vi "Generate XML String with Parser API.vi"() -> ()   [LabVIEW 2023]
doc: "This example illustrates how to create an XML document and save it as an XML file."
uses:
  <vilib>/Analysis/baseanly.llb/Mean (DBL).vi
  <vilib>/xml/Close Reference(Node).vi
  <resource>/objmgr/DOMUserDefRef.rc
  <vilib>/xml/NI_XML.lvlib
  <vilib>/Analysis/NI_AALBase.lvlib
panel:
  out "Generated XML":string
  # "Overview: Demonstrates the use of the XML Parser VIs and functions to generate an XML string that can adhere to an arbitrary schema.\nInstructions:\nRun the VI."
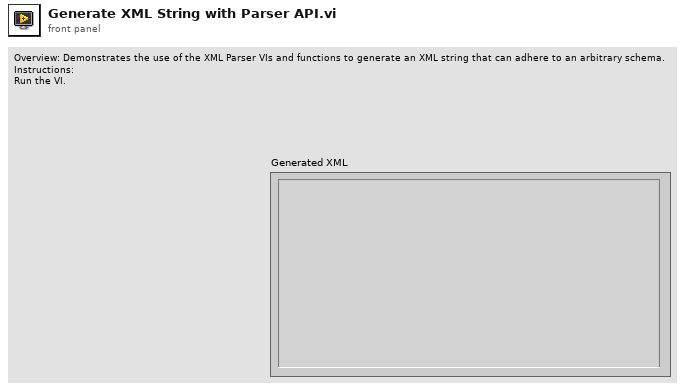
[diagram p1: front panel]
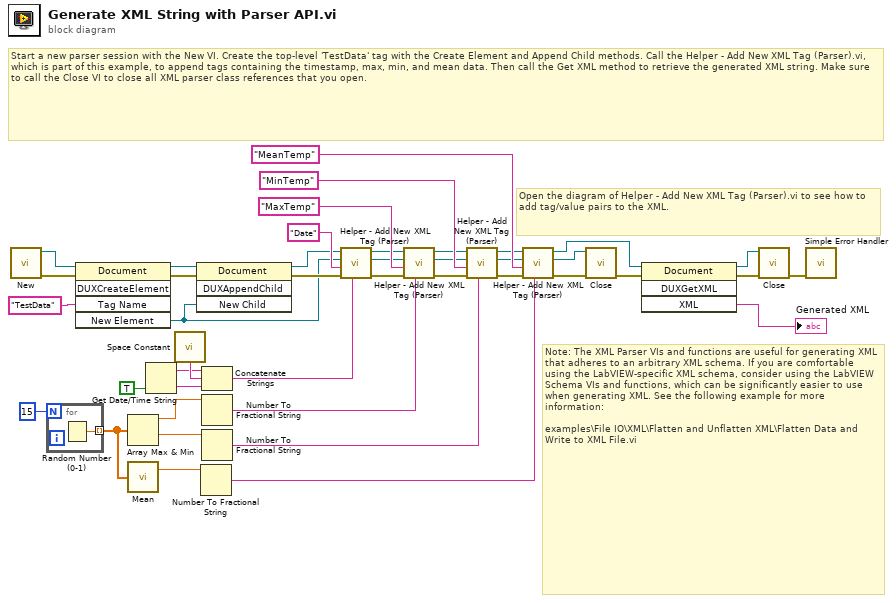
[diagram p0: block diagram]
diagram:
  # "Note: The XML Parser VIs and functions are useful for generating XML that adheres to an arbitrary XML schema. If you are comfortable using the LabVIEW-specific XML schema, consider using the LabVIEW Schema VIs and functions, which can be significantly easier to use when generating XML. See the following example for more information:\n\nexamples\\File IO\\XML\\Flatten and Unflatten XML\\Flatten Data and Write to XML File.vi"
  # "Open the diagram of Helper - Add New XML Tag (Parser).vi to see how to add tag/value pairs to the XML."
  # "Start a new parser session with the New VI. Create the top-level 'TestData' tag with the Create Element and Append Child methods. Call the Helper - Add New XML Tag (Parser).vi, which is part of this example, to append tags containing the timestamp, max, min, and mean data. Then call the Get XML method to retrieve the generated XML string. Make sure to call the Close VI to close all XML parser class references that you open."
  n1 = call <vilib>:"New.vi"() -> ("error out"=w29:errorcluster, "DOM document out"=w26:refnum<k20>)  [unwired: 1 in, 7 out]
  n2 = for {
    N: 15 -> [_]
    tunnel: [w43] -> w34 mode=indexing
    n3 = Random Number (0-1)() -> (number: 0 to 1=w43:dbl)
  }
  n4 = invoke class="Document" method="DUXCreateElement"(reference=w26, error in=w29, "Tag Name"="TestData" ("Qualified Name")) -> (reference out=w30:refnum<k20>, error out=w28:errorcluster, "New Element"=w5:refnum<k20>)  [unwired: 2 in, 2 out]
  n5 = Array Max & Min ("Max & Min")(array=w34) -> (max value=w1:dbl, min value=w2:dbl)  [unwired: 2 out]
  n6 = call-poly <vilib>:"Mean.vi"("X"=w34) -> ("mean"=w32:dbl)  [unwired: 1 out]
  n7 = Get Date/Time String(want seconds? (F)=TRUE) -> (date string=w40:string, time string=w39:string)  [unwired: 2 out]
  n8 = call <vilib>:"Space Constant.vi"() -> ("String"=w41:string)
  n9 = invoke class="Document" method="DUXAppendChild"(reference=w30, error in=w28, "New Child"=w5) -> (reference out=w9:refnum<k20>, error out=w7:errorcluster)  [unwired: 1 in, 2 out]
  n10 = Number To Fractional String(number=w32) -> (F-format string=w22:string)  [unwired: 3 out]
  n11 = Concatenate Strings(w40, w41, w39) -> (w3:string)
  n12 = Number To Fractional String(number=w1) -> (F-format string=w12:string)  [unwired: 3 out]
  n13 = Number To Fractional String(number=w2) -> (F-format string=w18:string)  [unwired: 3 out]
  n14 = call "Helper - Add New XML Tag (Parser).vi"("Tag Data"=w3, "error in (no error)"=w7, "Tag Name"="Date", "Owning Element"=w5, "DOM document"=w9) -> ("error out"=w6:errorcluster, "dup Owning Element"=w4:refnum<k20>, "dup DOM document"=w8:refnum<k20>)  [unwired: 4 in]
  n15 = call "Helper - Add New XML Tag (Parser).vi"("Tag Data"=w12, "error in (no error)"=w6, "Tag Name"="MaxTemp", "Owning Element"=w4, "DOM document"=w8) -> ("error out"=w15:errorcluster, "dup Owning Element"=w11:refnum<k20>, "dup DOM document"=w14:refnum<k20>)  [unwired: 4 in]
  n16 = call "Helper - Add New XML Tag (Parser).vi"("Tag Data"=w18, "error in (no error)"=w15, "Tag Name"="MinTemp", "Owning Element"=w11, "DOM document"=w14) -> ("error out"=w20:errorcluster, "dup Owning Element"=w19:refnum<k20>, "dup DOM document"=w16:refnum<k20>)  [unwired: 4 in]
  n17 = call "Helper - Add New XML Tag (Parser).vi"("Tag Data"=w22, "error in (no error)"=w20, "Tag Name"="MeanTemp", "Owning Element"=w19, "DOM document"=w16) -> ("error out"=w24:errorcluster, "dup Owning Element"=w21:refnum<k20>, "dup DOM document"=w23:refnum<k20>)  [unwired: 4 in]
  n18 = call-poly <vilib>:"Close.vi"("error in (no error)"=w24, "node"=w21) -> ("error out"=w35:errorcluster)  [unwired: 7 out]
  n19 = invoke class="Document" method="DUXGetXML"(reference=w23, error in=w35) -> (reference out=w36:refnum<k20>, error out=w38:errorcluster, "XML"=→"Generated XML":string)  [unwired: 2 in, 1 out]
  n20 = call-poly <vilib>:"Close.vi"("error in (no error)"=w38, "node"=w36) -> ("error out"=w27:errorcluster)  [unwired: 7 out]
  n21 = call <vilib>:"Simple Error Handler.vi"("error in (no error)"=w27) -> ()  [unwired: 1 in, 8 out]
